vi "Test MQTT-4.3.2-1.vi"(8 "error in (no error)":errorcluster, 11 "Connection Config":refnum<class "Connection.lvclass">) -> (0 "error out":errorcluster, 3 "Connection Config dup":refnum<class "Connection.lvclass">)   [LabVIEW 2013]
uses:
  <vilib>/LabVIEW Open Source Project/MQTT Control Packets/Control Packets/CONNECT/CONNECT.lvclass
  <vilib>/LabVIEW Open Source Project/MQTT Control Packets/Control Packets/ControlPacket/ControlPacket.lvclass
  <vilib>/addons/_JKI Toolkits/Caraya/classes/Test/Test.lvclass
  <vilib>/LabVIEW Open Source Project/MQTT Control Packets/Control Packets/DISCONNECT/DISCONNECT.lvclass
  <vilib>/LabVIEW Open Source Project/Connection/Connection/Connection.lvclass
  <vilib>/LabVIEW Open Source Project/MQTT Control Packets/Control Packets/SUBSCRIBE/SUBSCRIBE.lvclass
  <vilib>/LabVIEW Open Source Project/MQTT Control Packets/Control Packets/ControlPacket/QualityOfService -- enum.ctl
  <vilib>/LabVIEW Open Source Project/MQTT Control Packets/Control Packets/SUBSCRIBE/Topic Subscription -- cluster.ctl
  <vilib>/LabVIEW Open Source Project/MQTT Control Packets/Control Packets/PUBLISH/PUBLISH.lvclass
  <vilib>/addons/_JKI Toolkits/Caraya/classes/Assert/Assert.lvclass
  <vilib>/addons/_JKI Toolkits/Caraya/classes/Assert/Assert True.vi
  <vilib>/LabVIEW Open Source Project/MQTT Connection/MQTT_Connection/Connection/Connection.lvclass
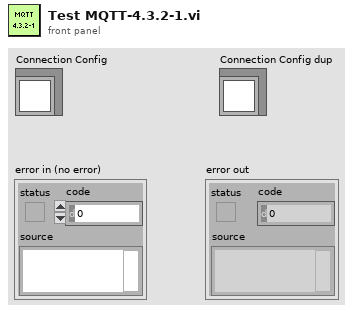
[diagram p1: front panel]
types:
  T1 = typedef "MQTT_Control_Packets.lvlib/ControlPacket.lvclass/QualityOfService -- enum.ctl" = enum16{"0 (At Most Once)", "1 (At Least Once)", "2 (Exactly Once)"}
  T2 = typedef "MQTT_Control_Packets.lvlib/SUBSCRIBE.lvclass/Topic Subscription -- cluster.ctl" = cluster{"Topic Filter":string, "QoS":T1}
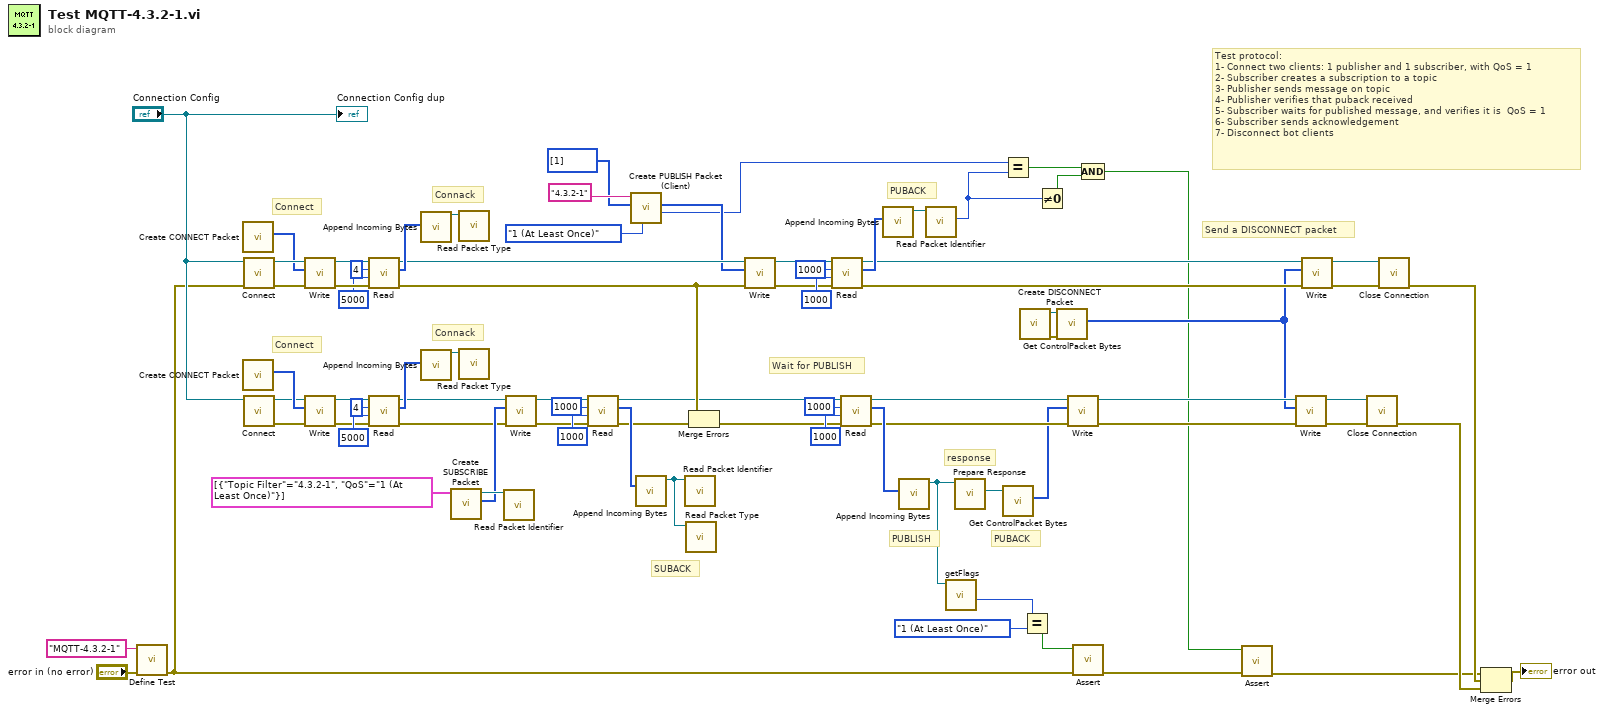
[diagram p0: block diagram]
diagram:
  # "response"
  # "PUBACK"
  # "PUBLISH"
  # "Wait for PUBLISH"
  # "PUBACK"
  # "SUBACK"
  # "Connack"
  # "Connect"
  # "Connack"
  # "Connect"
  # "Test protocol: \n1- Connect two clients: 1 publisher and 1 subscriber, with QoS = 1\n2- Subscriber creates a subscription to a topic\n3- Publisher sends message on topic\n4- Publisher verifies that puback received\n5- Subscriber waits for published message, and verifies it is  QoS = 1\n6- Subscriber sends acknowledgement\n7- Disconnect bot clients"
  # "Send a DISCONNECT packet"
  n1 = call <vilib>:"Define Test.vi"("error in (no error)"="error in (no error)", "Label (VI Title)"="MQTT-4.3.2-1") -> ("error out"=w8:errorcluster)  [unwired: 9 in]
  n2 = call <vilib>:"Create CONNECT Packet.vi"() -> ("Bytes Stream"=w68:u8[])  [unwired: 9 in, 2 out]
  n3 = call <vilib>:"Create CONNECT Packet.vi"() -> ("Bytes Stream"=w62:u8[])  [unwired: 9 in, 2 out]
  n4 = call <vilib>:"Connect.vi"("error in (no error)"=w8, "Connection in"="Connection Config") -> ("error out"=w72:errorcluster, "Connection out"=w71:refnum<class "Connection.lvclass">)  [unwired: 8 in]
  n5 = call <vilib>:"Connect.vi"("Connection in"="Connection Config") -> ("error out"=w59:errorcluster, "Connection out"=w60:refnum<class "Connection.lvclass">)  [unwired: 9 in]
  n6 = call <vilib>:"Write.vi"("error in (no error)"=w72, "Bytes"=w68, "Connection in"=w71) -> ("error out"=w73:errorcluster, "Connection"=w74:refnum<class "Connection.lvclass">)  [unwired: 7 in]
  n7 = call <vilib>:"Write.vi"("error in (no error)"=w59, "Bytes"=w62, "Connection in"=w60) -> ("error out"=w58:errorcluster, "Connection"=w57:refnum<class "Connection.lvclass">)  [unwired: 7 in]
  n8 = call <vilib>:"Read.vi"("error in (no error)"=w73, "timeout (2000 ms)"=5000 ("timeout (1000 ms)"), "bytes to read (100)"=4 ("bytes to read"), "TCPConnection in"=w74) -> ("error out"=w39:errorcluster, "Bytes"=w67:u8[], "TCPConnection out"=w38:refnum<class "Connection.lvclass">)  [unwired: 3 in, 2 out]
  n9 = call <vilib>:"Read.vi"("error in (no error)"=w58, "timeout (2000 ms)"=5000 ("timeout (1000 ms)"), "bytes to read (100)"=4 ("bytes to read"), "TCPConnection in"=w57) -> ("error out"=w50:errorcluster, "Bytes"=w63:u8[], "TCPConnection out"=w52:refnum<class "Connection.lvclass">)  [unwired: 3 in, 2 out]
  n10 = call <vilib>:"Append Incoming Bytes.vi"("Incoming Packets"=w67) -> ("ControlPacket"=w66:refnum<class "ControlPacket.lvclass">)  [unwired: 7 in, 3 out]
  n11 = call <vilib>:"Append Incoming Bytes.vi"("Incoming Packets"=w63) -> ("ControlPacket"=w64:refnum<class "ControlPacket.lvclass">)  [unwired: 7 in, 3 out]
  n12 = call <vilib>:"Create SUBSCRIBE Packet.vi"("Topic Subscriptions"=T2[] [{"Topic Filter"="4.3.2-1", "QoS"=enum."1 (At Least Once)"}]) -> ("Bytes Stream"=w51:u8[], "SUBSCRIBE out"=w53:refnum<class "SUBSCRIBE.lvclass">)  [unwired: 8 in, 1 out]
  n13 = call <vilib>:"Read Packet Type.vi"("ControlPacket in"=w66) -> ()  [unwired: 9 in, 2 out]
  n14 = call <vilib>:"Read Packet Type.vi"("ControlPacket in"=w64) -> ()  [unwired: 9 in, 2 out]
  n15 = call <vilib>:"Read Packet Identifier.vi"("ControlPacket in"=w53) -> ()  [unwired: 9 in, 2 out]
  n16 = call <vilib>:"Write.vi"("error in (no error)"=w50, "Bytes"=w51, "Connection in"=w52) -> ("error out"=w46:errorcluster, "Connection"=w47:refnum<class "Connection.lvclass">)  [unwired: 7 in]
  n17 = call <vilib>:"Read.vi"("error in (no error)"=w46, "timeout (2000 ms)"=1000 ("timeout (1000 ms)"), "bytes to read (100)"=1000 ("bytes to read"), "TCPConnection in"=w47) -> ("error out"=w43:errorcluster, "Bytes"=w45:u8[], "TCPConnection out"=w25:refnum<class "Connection.lvclass">)  [unwired: 3 in, 2 out]
  n18 = call <vilib>:"Create PUBLISH Packet (Client).vi"("QoS"=QualityOfService_--_enum."1 (At Least Once)", "Payload"=u8[] [1], "Topic Name"="4.3.2-1" ("Topic Filter")) -> ("Packet ID"=w6:u16, "Bytes Stream"=w37:u8[])  [unwired: 5 in, 2 out]
  n19 = call <vilib>:"Append Incoming Bytes.vi"("Incoming Packets"=w45) -> ("ControlPacket"=w44:refnum<class "ControlPacket.lvclass">)  [unwired: 7 in, 3 out]
  n20 = call <vilib>:"Read Packet Identifier.vi"("ControlPacket in"=w44) -> ()  [unwired: 9 in, 2 out]
  n21 = call <vilib>:"Read Packet Type.vi"("ControlPacket in"=w44) -> ()  [unwired: 9 in, 2 out]
  n22 = Merge Errors(w39, w43) -> (w24:errorcluster)
  n23 = call <vilib>:"Write.vi"("error in (no error)"=w39, "Bytes"=w37, "Connection in"=w38) -> ("error out"=w31:errorcluster, "Connection"=w33:refnum<class "Connection.lvclass">)  [unwired: 7 in]
  n24 = call <vilib>:"Read.vi"("error in (no error)"=w31, "timeout (2000 ms)"=1000 ("timeout (1000 ms)"), "bytes to read (100)"=1000 ("bytes to read"), "TCPConnection in"=w33) -> ("error out"=w30:errorcluster, "Bytes"=w36:u8[], "TCPConnection out"=w32:refnum<class "Connection.lvclass">)  [unwired: 3 in, 2 out]
  n25 = call <vilib>:"Read.vi"("error in (no error)"=w24, "timeout (2000 ms)"=1000 ("timeout (1000 ms)"), "bytes to read (100)"=1000 ("bytes to read"), "TCPConnection in"=w25) -> ("error out"=w22:errorcluster, "Bytes"=w28:u8[], "TCPConnection out"=w23:refnum<class "Connection.lvclass">)  [unwired: 3 in, 2 out]
  n26 = call <vilib>:"Append Incoming Bytes.vi"("Incoming Packets"=w36) -> ("ControlPacket"=w29:refnum<class "ControlPacket.lvclass">)  [unwired: 7 in, 3 out]
  n27 = call <vilib>:"Append Incoming Bytes.vi"("Incoming Packets"=w28) -> ("ControlPacket"=w19:refnum<class "ControlPacket.lvclass">)  [unwired: 7 in, 3 out]
  n28 = call <vilib>:"Read Packet Identifier.vi"("ControlPacket in"=w29) -> ("Packet Identifier"=w4:u16)  [unwired: 9 in, 1 out]
  n29 = call-dynamic "getFlags.vi"("ControlPacket in"=w19) -> ("QoS"=w18:T1)  [unwired: 7 in, 3 out]
  n30 = call-dynamic "Prepare Response.vi"("ControlPacket in"=w19) -> ("ControlPacket response"=w21:refnum<class "ControlPacket.lvclass">)  [unwired: 7 in, 3 out]
  n31 = Equal?(x=w6, y=w4) -> (x = y?=w2:bool)
  n32 = call <vilib>:"Get ControlPacket Bytes.vi"("ControlPacket"=w21) -> ("Bytes Stream"=w20:u8[])  [unwired: 7 in, 3 out]
  n33 = call <vilib>:"Create DISCONNECT Packet.vi"() -> ("error out"=w77:errorcluster, "DISCONNECT"=w76:refnum<class "DISCONNECT.lvclass">)  [unwired: 9 in, 1 out]
  n34 = Equal?(x=w18, y=QualityOfService_--_enum."1 (At Least Once)") -> (x = y?=w9:bool)
  n35 = Not Equal To 0?(x=w4) -> (x != 0?=w3:bool)
  n36 = call <vilib>:"Get ControlPacket Bytes.vi"("error in (no error)"=w77, "ControlPacket"=w76) -> ("Bytes Stream"=w13:u8[])  [unwired: 6 in, 3 out]
  n37 = call <vilib>:"Write.vi"("error in (no error)"=w22, "Bytes"=w20, "Connection in"=w23) -> ("error out"=w15:errorcluster, "Connection"=w16:refnum<class "Connection.lvclass">)  [unwired: 7 in]
  n38 = call-poly <vilib>:"Assert.vi"("error in (no error)"=w8, "True?"=w9) -> ("error out"=w7:errorcluster)  [unwired: 9 in]
  n39 = Compound Arithmetic op=AND(w2, w3) -> (w1:bool)
  n40 = call-poly <vilib>:"Assert.vi"("error in (no error)"=w7, "True?"=w1) -> ("error out"=w5:errorcluster)  [unwired: 9 in]
  n41 = call <vilib>:"Write.vi"("error in (no error)"=w15, "Bytes"=w13, "Connection in"=w16) -> ("error out"=w11:errorcluster, "Connection"=w12:refnum<class "Connection.lvclass">)  [unwired: 7 in]
  n42 = call <vilib>:"Write.vi"("error in (no error)"=w30, "Bytes"=w13, "Connection in"=w32) -> ("error out"=w14:errorcluster, "Connection"=w70:refnum<class "Connection.lvclass">)  [unwired: 7 in]
  n43 = call <vilib>:"Close Connection.vi"("error in (no error)"=w11, "Connection in"=w12) -> ("error out"=w10:errorcluster)  [unwired: 8 in, 1 out]
  n44 = call <vilib>:"Close Connection.vi"("error in (no error)"=w14, "Connection in"=w70) -> ("error out"=w65:errorcluster)  [unwired: 8 in, 1 out]
  n45 = Merge Errors(w5, w65, w10) -> (→"error out":errorcluster)
  "Connection Config dup" <- "Connection Config"
